vi "USB9825_DI.vi"(8 "错误输入（无错误）":errorcluster, 11 "hDevice":i32) -> (0 "错误输出":errorcluster, 3 "pDI":i32)   [LabVIEW 2015, in "DAQ.lvlib"]
uses:
  DAQ.lvlib
  USB9825.DLL
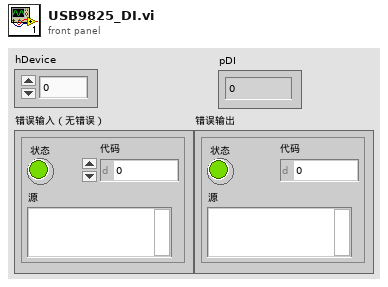
[diagram p1: front panel]
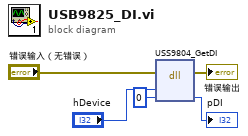
[diagram p0: block diagram]
diagram:
  n1 = dll-call lib="PTH2sabs CYexinrongWorkplace\t普密斯Thickness-measurementBiometry_alpha3 bolihouduSub VIsDAQUSB9825.dll" fn="USS9804_GetDI"(error in="错误输入（无错误）", "hDevice"="hDevice", "pDI"=0) -> (error out=→"错误输出":errorcluster, "pDI"=→"pDI":i32)  [unwired: 4 in, 1 out]
